vi "Write Splitter Refnum.vi"(8 "error in (no error)":errorcluster, 10 "Splitter Refnum":refnum<vi>, 11 "Docking in":refnum<class "Docking.lvclass">) -> (0 "error out":errorcluster, 3 "Docking out":refnum<class "Docking.lvclass">)   [LabVIEW 2023, in "Docking.lvlib" / "Docking.lvclass"]
doc: "Writes the splitter refnum to private data for access/update.\nWhen writing the splitter refnum, this routine also reads the initial position of the splitter and stores the initial position to private data."
uses:
  Docking.lvclass
  Docking.lvclass/Docking.ctl
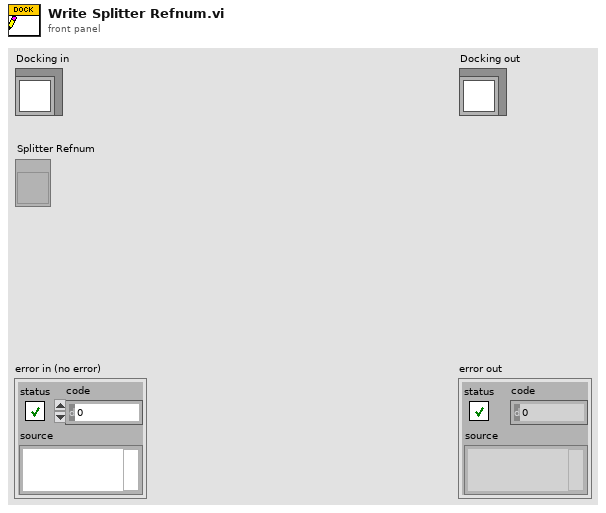
[diagram p1: front panel]
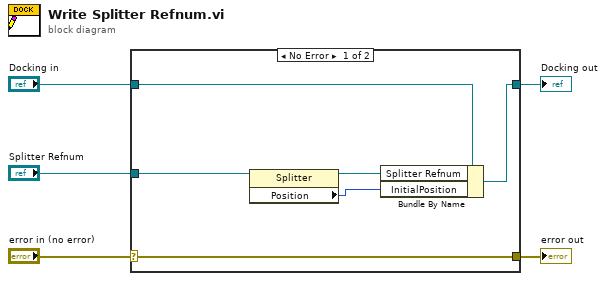
[diagram p0: block diagram]
diagram:
  n1 = case shown="No Error" "error in (no error)" {
    selector: "error in (no error)" -> [w11 w12]
    tunnel: [w11 w12] -> w4
    tunnel: [w9 w13] -> w2
    tunnel: "Docking in" -> [w10 w13]
    tunnel: "Splitter Refnum" -> [w8 _]
    frame No Error {
      n2 = property class="Splitter"(reference=w8) -> (reference out=w7:refnum<vi>, "Position"=w6:i32)  [unwired: 1 in, 1 out]
      n3 = Bundle By Name(cluster=w10, "Splitter Refnum"=w7, "InitialPosition"=w6) -> (w9:refnum<class "Docking.lvclass">)
    }
    frame Error {
    }
  }
  "error out" <- w4
  "Docking out" <- w2
